vi "V7310.Main-Print.vi"(8 "error in":errorcluster, 10 "Slot":T9, 11 "Code sets in":T2={"Ready"=FALSE, "DoubleOrder"=FALSE, "OrderDone"=FALSE, "AllowSingleSlot"=FALSE, "CheckDM"=FALSE, "ThresholdA"=0, "ThresholdB"=0, "Plate"=enum."Wabco", "ImgPath"=path "", "Variant"={"State"=enum."Init", "ImgPath"=path "", "WabcoPlate"="", "WabcoProduct"="", "ClientProduct"="", "ClientPlate"="", "TotalQuantity"=0, "OrderQuantity"=0, "Serial"=0, "Wabco"={"LaserJob"="", "AdditionalTxt"="037", "FactoryCode"="", "RevID"=0, "ForkID"=0, "FailuresLimit"=0, "GlobalCnt"=0, "Bank"=0, "SerialFormat"=enum."6 dig", "CoordA"={"X"=0.0, "Y"=0.0, "Angle"=0.0}, "CoordB"={"X"=0.0, "Y"=0.0, "Angle"=0.0}, "DMCconfig"=0}, "Client"={"LaserJob"="", "AdditionalTxt"="", "FactoryCode"="037", "RevID"=0, "ForkID"=0, "FailuresLimit"=0, "GlobalCnt"=0, "Bank"=0, "SerialFormat"=enum."6 dig", "CoordA"={"X"=0.0, "Y"=0.0, "Angle"=0.0}, "CoordB"={"X"=0.0, "Y"=0.0, "Angle"=0.0}, "DMCconfig"=0}}}) -> (0 "error out":errorcluster, 1 "Status":T1, 2 "Aborted":bool, 3 "Serial":i32, 5 "LaserVars":string[](array[string]))   [LabVIEW 2016]
uses:
  Station/Station.ProductSlot.ctl
  Sequence/Sequence.Code.Sets.ctl
  Sequence/Sequence.PlateType.ctl
  Logger/Logger.Variant.Sets.ctl
  Station/Station.Changeover.State.vi
  Station/Station.Plate.Properties.ctl
  Sequence/Sequence.Code.SerialFormat.ctl
  LowLevel/V7310.Job.Sets.ctl
  Sequence/Sequence.Step.Status.ctl
  LowLevel/V7310.Job.Data.ctl
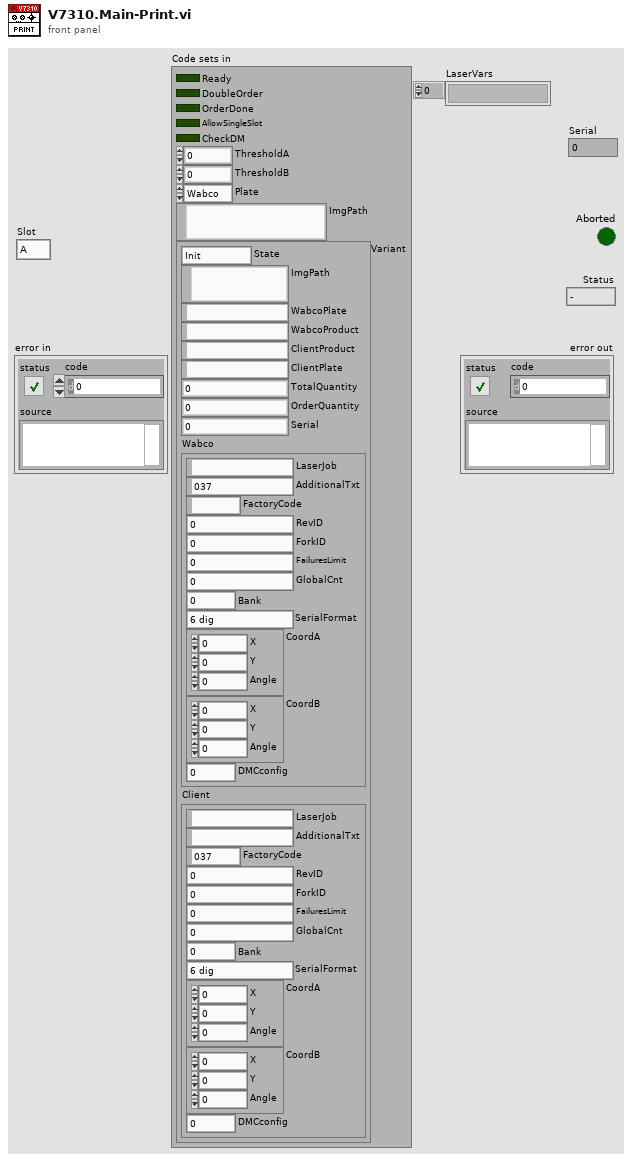
[diagram p1: front panel]
types:
  T1 = typedef "Sequence.Step.Status.ctl" = enum16{"-", "Pending", "Running", "Skipped", "Passed", "Failed", "Done", "Error", "Aborted", "Stopped"}
  T2 = typedef "Sequence.Code.Sets.ctl" = cluster{"Ready":bool, "DoubleOrder":bool, "OrderDone":bool, "AllowSingleSlot":bool, "CheckDM":bool, "ThresholdA":u8, "ThresholdB":u8, "Plate":T3, "ImgPath":path, "Variant":T4}
  T3 = typedef "Sequence.PlateType.ctl" = enum16{"Wabco", "Client"}
  T4 = typedef "Logger.Variant.Sets.ctl" = cluster{"State":T5, "ImgPath":path, "WabcoPlate":string, "WabcoProduct":string, "ClientProduct":string, "ClientPlate":string, "TotalQuantity":u16, "OrderQuantity":u16, "Serial":i32, "Wabco":T6, "Client":T6}
  T5 = typedef "Station.Changeover.State.vi" = enum16{"Init", "Scaning", "NOK", "Wait for ack", "Ready"}
  T6 = typedef "Station.Plate.Properties.ctl" = cluster{"LaserJob":string, "AdditionalTxt":string, "FactoryCode":string, "RevID":u8, "ForkID":u8, "FailuresLimit":u16, "GlobalCnt":i32, "Bank":u8, "SerialFormat":T7, "CoordA":T8, "CoordB":T8, "DMCconfig":i32}
  T7 = typedef "Sequence.Code.SerialFormat.ctl" = enum8{"", "6 dig", "7 dig"}
  T8 = typedef "V7310.Job.Sets.ctl" = cluster{"X":dbl, "Y":dbl, "Angle":dbl}
  T9 = typedef "Station.ProductSlot.ctl" = enum8{"A", "B"}
  T10 = typedef "V7310.Job.Data.ctl" = cluster{"Vars":string[], "Sets":T8}
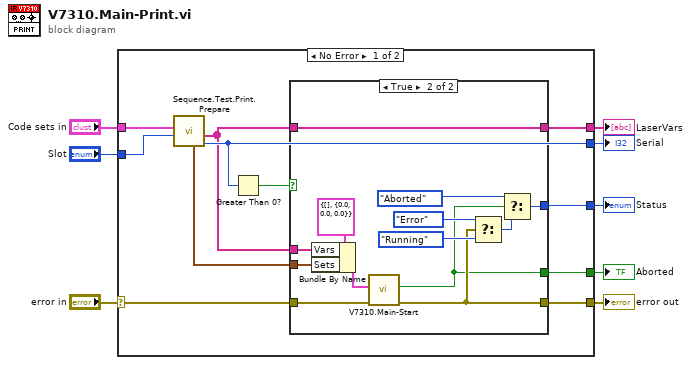
[diagram p0: block diagram]
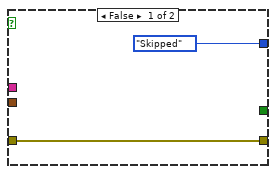
[diagram p2: hidden frame]
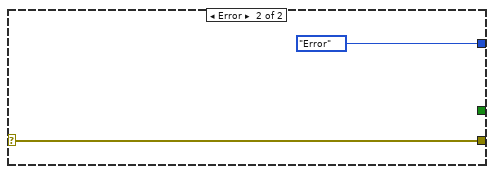
[diagram p3: hidden frame]
diagram:
  n1 = case shown="No Error" "error in" {
    selector: "error in" -> [w12 w36]
    tunnel: [w11 w36] -> w7
    tunnel: [w19 _] -> w6
    tunnel: "Code sets in" -> [w16 _]
    tunnel: [w18 Sequence.Step.Status."Error" ("status")] -> w4
    tunnel: "Slot" -> [w14 _]
    tunnel: [w10 _] -> w1
    tunnel: [w15 _] -> w2
    frame No Error {
      n2 = call "Sequence.Test.Print.Prepare.vi"("Slot"=w14, "Code sets in"=w16) -> ("NextSerial"=w15:i32, "Variables"=w9:string[], "JobSets"=w13:T8)  [unwired: 7 in]
      n3 = Greater Than 0?(x=w15) -> (x > 0?=w17:bool)
      n4 = case shown="True" w17 {
        tunnel: w12 -> [w20 w34]
        tunnel: [w20 w25] -> w11
        tunnel: [_ w23] -> w19
        tunnel: [Sequence.Step.Status."Skipped" ("status") w33] -> w18
        tunnel: w13 -> [_ w32]
        tunnel: w9 -> [_ w24]
        tunnel: w9 -> [_ w22]
        tunnel: [_ w22] -> w10
        frame False {
        }
        frame True {
          n5 = Bundle By Name(cluster=T10 {"Vars"=[], "Sets"={"X"=0.0, "Y"=0.0, "Angle"=0.0}} ("Job"), "Vars"=w24, "Sets"=w32) -> (w26:T10)
          n6 = call "V7310.Main-Start.vi"("error in"=w34, "Job"=w26) -> ("error out"=w25:errorcluster, "Aborted"=w23:bool)  [unwired: 8 in]
          n7 = Select(t=Sequence.Step.Status."Error" ("status"), s=w25, f=Sequence.Step.Status."Running" ("status")) -> (s? t:f=w31:T1)
          n8 = Select(t=Sequence.Step.Status."Aborted" ("status"), s=w23, f=w31) -> (s? t:f=w33:T1)
        }
      }
    }
    frame Error {
    }
  }
  "error out" <- w7
  "Aborted" <- w6
  "Status" <- w4
  "Serial" <- w2
  "LaserVars" <- w1
